vi "RD Digital I2C Rx.vi"(0 "handle":u64, 1 "rxcount":i32, 5 "addr":u8, 9 "length":i32, 11 "error in (no error)":errorcluster caption="错误输入（无错误）", 12 "fParity":i32) -> (3 "rxcount out":i32, 4 "handle out":u64, 6 "function return":i32, 8 "rgRX out":u8[](array[numeric]), 14 "fParity out":i32, 15 "error out":errorcluster caption="错误输出")   [LabVIEW 2018, in "InstrumentsPlayground.lvlib"]
doc: "CLIFFAPI int CliffDigitalI2CRx(FT_HANDLE handle,uchar addr, uchar* rgRX, int length, int * rxcount, int *fParity);"
uses:
  InstrumentsPlayground.lvlib
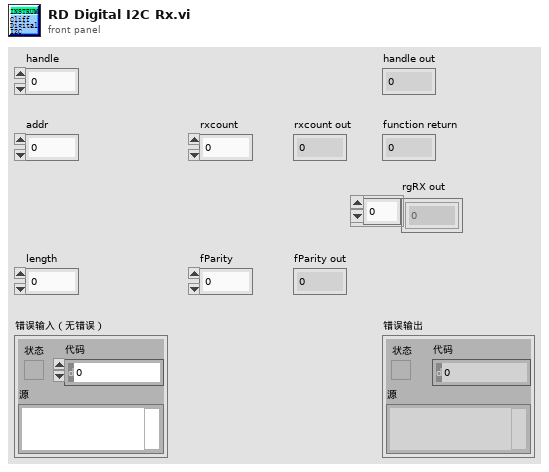
[diagram p1: front panel]
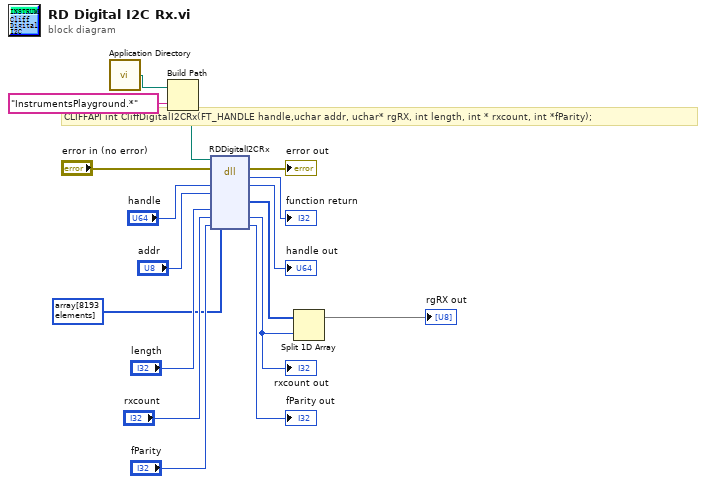
[diagram p0: block diagram]
diagram:
  # "CLIFFAPI int CliffDigitalI2CRx(FT_HANDLE handle,uchar addr, uchar* rgRX, int length, int * rxcount, int *fParity);"
  n1 = call <vilib>:"Application Directory.vi"() -> ("Application Directory"=w5:path)
  n2 = Build Path(base path=w5, name or relative path="InstrumentsPlayground.*" ("名称或相对路径")) -> (appended path=w4:path)
  n3 = dll-call lib="E:/Work/YZCourse_Xtext/Cliff/API/IPLabView lib/InstrumentsPlayground.*" fn="RDDigitalI2CRx"(path in=w4, error in="error in (no error)", "handle"="handle", "addr"="addr", "rgRX"=u8[] array[8193 elements], "length"="length", "rxcount"="rxcount", "fParity"="fParity") -> (error out=→"error out":errorcluster, "返回类型"=→"function return":i32, "handle"=→"handle out":u32, "rgRX"=w13:u8[], "rxcount"=w2:i32, "fParity"=→"fParity out":i32)  [unwired: 3 in, 1 out]
  "rxcount out" <- w2
  n4 = Split 1D Array(array=w13, index=w2) -> (first subarray=→"rgRX out":u8[])  [unwired: 1 out]
